vi "Create Policy Version.vi"(6 "Set as Default":bool=TRUE, 8 "error in (no error)":errorcluster, 9 "Policy JSON":string, 10 "Name":string, 11 "IoT Session in":refnum<class "IoT Session.lvclass">) -> (0 "error out":errorcluster, 3 "IoT Session out":refnum<class "IoT Session.lvclass">)   [LabVIEW 2015, in "NI_AWS_IoT.lvlib" / "IoT Session.lvclass"]
uses:
  IoT Session.lvclass
  Core/HTTP Request/Valid String Specification.ctl
  Core/HTTP Request/Request Options.ctl
  Core/HTTP Request/Name Value Pair.ctl
  Core/HTTP Request/Region handling.ctl
  Core/HTTP Request/URL formatting.ctl
  Core/HTTP Request/HTTP Request.lvclass
  JSON Parsing/NI_JSON Parsing.lvlib
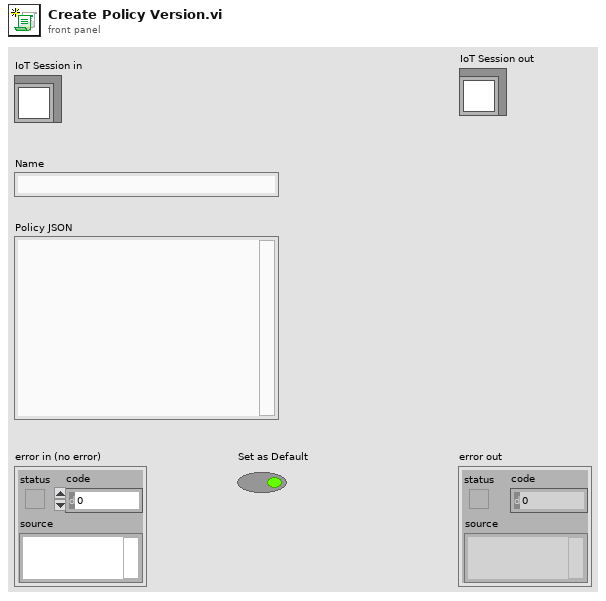
[diagram p1: front panel]
types:
  T1 = typedef "NI_AWS_Core.lvlib/HTTP Request.lvclass/Valid String Specification.ctl" = enum16{"none", "only [alphanumeric][-][_]", "only [alphanumeric][-][_][space]", "phone number +1xxxyyyzzzz", "Regular Expression"}
  T2 = typedef "NI_AWS_Core.lvlib/HTTP Request.lvclass/Name Value Pair.ctl" = cluster{"name":string, "value":string}
  T3 = typedef "NI_AWS_Core.lvlib/HTTP Request.lvclass/Request Options.ctl" = cluster{"request headers":T2[], "request parameters":T2[], "request body":string, "region handling":T4, "URL formatting":T5}
  T4 = typedef "NI_AWS_Core.lvlib/HTTP Request.lvclass/Region handling.ctl" = enum16{"use region everywhere", "use region (authentication only)", "use region (URL only)", "ignore region everwhere"}
  T5 = typedef "NI_AWS_Core.lvlib/HTTP Request.lvclass/URL formatting.ctl" = enum16{"region-", "region."}
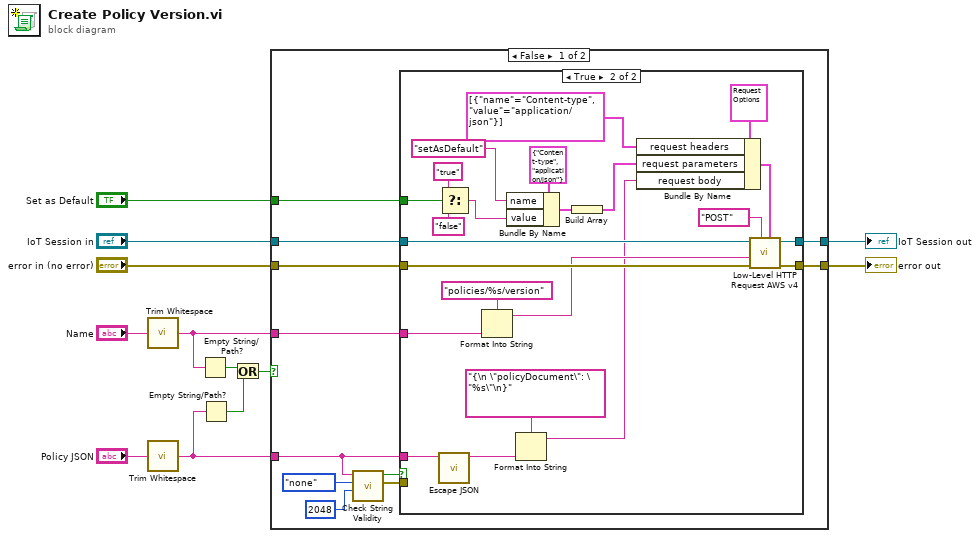
[diagram p0: block diagram]
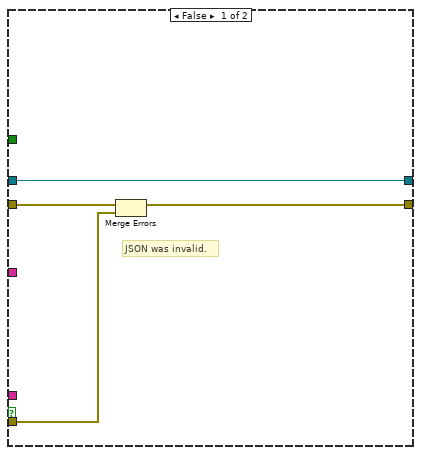
[diagram p2: hidden frame]
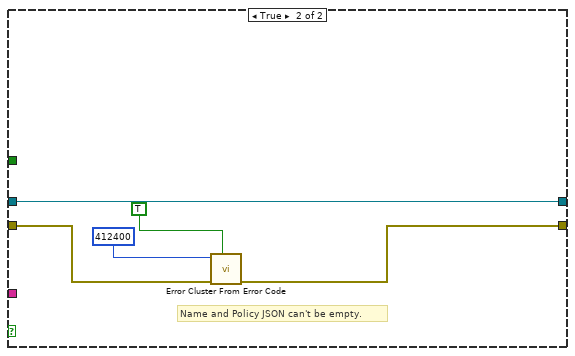
[diagram p3: hidden frame]
diagram:
  n1 = call <vilib>:"Trim Whitespace.vi"("string"="Name") -> ("trimmed string"=w6:string)  [unwired: 1 in]
  n2 = call <vilib>:"Trim Whitespace.vi"("string"="Policy JSON") -> ("trimmed string"=w5:string)  [unwired: 1 in]
  n3 = Empty String/Path?(string/path=w6) -> (empty?=w4:bool)
  n4 = Empty String/Path?(string/path=w5) -> (empty?=w3:bool)
  n5 = Or(x=w4, y=w3) -> (x .or. y?=w2:bool)
  n6 = case shown="False" w2 {
    tunnel: "error in (no error)" -> [w23 w55]
    tunnel: [w22 w54] -> w11
    tunnel: [w21 w52] -> w10
    tunnel: w5 -> [w16 _]
    tunnel: "IoT Session in" -> [w20 w52]
    tunnel: w6 -> [w19 _]
    tunnel: "Set as Default" -> [w13 _]
    frame False {
      n7 = call "Check String Validity.vi"("Max Characters"=2048, "Valid String Specification"=Valid_String_Specification."none", "String"=w16) -> ("string error"=w15:errorcluster, "Valid"=w14:bool)  [unwired: 7 in]
      n8 = case shown="True" w14 {
        tunnel: w23 -> [w27 w50]
        tunnel: [w26 w49] -> w22
        tunnel: [w25 w48] -> w21
        tunnel: w19 -> [_ w44]
        tunnel: w20 -> [w25 w41]
        tunnel: w16 -> [_ w38]
        tunnel: w15 -> [w24 _]
        tunnel: w13 -> [_ w35]
        frame False {
          # "JSON was invalid."
          n9 = Merge Errors(w27, w24) -> (w26:errorcluster)
        }
        frame True {
          n10 = call "Escape JSON.vi"("JSON"=w38) -> ("Escaped JSON"=w37:string)  [unwired: 10 in]
          n11 = Select(t="true", s=w35, f="false") -> (s? t:f=w29:string)
          n12 = Format Into String(format string="policies/%s/version", w44) -> (resulting string=w45:string)  [unwired: 2 in, 1 out]
          n13 = Bundle By Name(cluster=T2 {"name"="Content-type", "value"="application/json"} ("Cluster"), "name"="setAsDefault", "value"=w29) -> (w31:T2)
          n14 = Format Into String(format string="{\n \"policyDocument\": \"%s\"\n}", w37) -> (resulting string=w39:string)  [unwired: 2 in, 1 out]
          n15 = Build Array(w31) -> (w30:T2[])
          n16 = Bundle By Name(cluster=T3 {"request headers"=[], "request parameters"=[], "request body"="", "region handling"=enum."use region everywhere", "URL formatting"=enum."region."} ("Request Options"), "request headers"=T2[] [{"name"="Content-type", "value"="application/json"}], "request parameters"=w30, "request body"=w39) -> (w42:T3)
          n17 = call "Low-Level HTTP Request AWS v4.vi"("Request Options"=w42, "HTTP-Verb"="POST", "error in (no error)"=w50, "URL Suffix"=w45, "AWS Core in"=w41) -> ("error out"=w49:errorcluster, "AWS Core out"=w48:refnum<class "IoT Session.lvclass">)  [unwired: 3 in, 2 out]
        }
      }
    }
    frame True {
      # "Name and Policy JSON can't be empty."
      n18 = call <vilib>:"Error Cluster From Error Code.vi"("show call chain? (False)"=TRUE, "error in (no error)"=w55, "error code (0)"=412400) -> ("error out"=w54:errorcluster)  [unwired: 6 in]
    }
  }
  "error out" <- w11
  "IoT Session out" <- w10
